vi "Convert From JSON Comp Format.vi"(8 "error in (no error)":errorcluster, 11 "input settings JSON":T1={"number of channels"=51200, "data justification"="", "endianness"="", "channel length"=5, "bit depth"=0, "frame clock rate"=0.0, "bit clock edge sync"="", "master clock souce"="", "master clock rate"=0.0, "logic level"="", "frame sync edge for channel 0"="", "Channel 0 Offset"=0}) -> (0 "error out":errorcluster, 3 "input settings":T2={"number of channels"=51200, "data justification"=enum."Right Justified", "endianness"=enum."MSB First", "channel length"=0, "bit depth"=0, "frame clock rate"=0.0, "bit clock edge sync"=enum."Falling", "master clock source"=enum."Internal", "master clock rate"=0.0, "Logic Level"=enum."1.2 V", "frame sync edge for channel 0"=enum."Rising", "Channel 0 Offset"=0})   [LabVIEW 2022 SP3, in "Digital Serial Input Settings.lvlib"]
uses:
  Digital Serial Input Settings.lvlib
  controls/digital serial input settings.ctl
  <vilib>/PDM Acquisition Toolkit/shared/controls/PCM Data Justification.ctl
  <vilib>/PDM Acquisition Toolkit/shared/controls/PCM Bit Endianness.ctl
  <vilib>/PDM Acquisition Toolkit/shared/controls/Digital Edge.ctl
  controls/digital audio protocol/master clock source.ctl
  <vilib>/PDM Acquisition Toolkit/host/Classes/Session/Controls/Logic Levels.ctl
  digital serial input settings_json.ctl
  <vilib>/PDM Acquisition Toolkit/shared/PDM Shared.lvlib
  <vilib>/PDM Acquisition Toolkit/host/Classes/Session/DecoderSession.lvclass
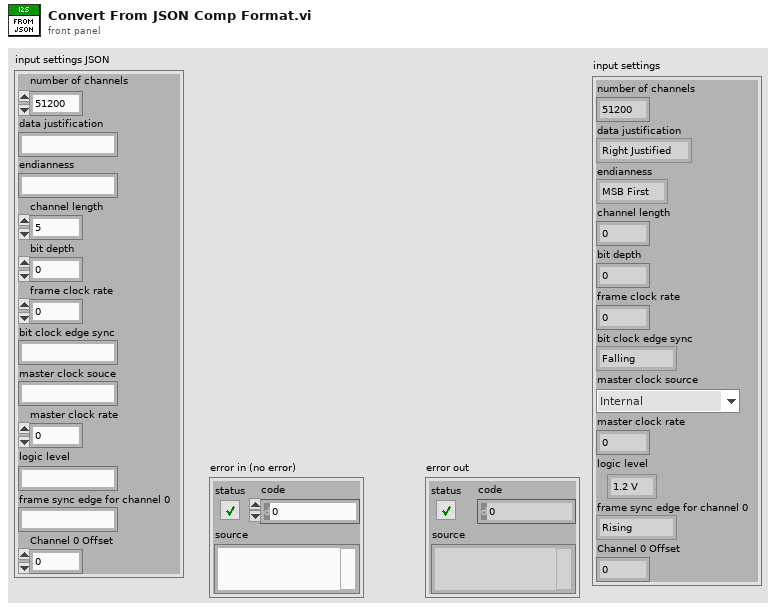
[diagram p1: front panel]
types:
  T1 = typedef "Digital Serial Input Settings.lvlib/digital serial input settings_json.ctl" = cluster{"number of channels":u32, "data justification":string, "endianness":string, "channel length":u32, "bit depth":u32, "frame clock rate":dbl, "bit clock edge sync":string, "master clock souce":string, "master clock rate":dbl, "logic level":string, "frame sync edge for channel 0":string, "Channel 0 Offset":u32}
  T2 = typedef "digital serial input settings.ctl" = cluster{"number of channels":u32, "data justification":T3, "endianness":T4, "channel length":u32, "bit depth":u32, "frame clock rate":dbl, "bit clock edge sync":T5, "master clock source":T6, "master clock rate":dbl, "Logic Level":T7, "frame sync edge for channel 0":T5, "Channel 0 Offset":u32}
  T3 = typedef "PDM Shared.lvlib/PCM Data Justification.ctl" = enum16{"Left Justified", "Right Justified"}
  T4 = typedef "PDM Shared.lvlib/PCM Bit Endianness.ctl" = enum16{"MSB First", "LSB First"}
  T5 = typedef "PDM Shared.lvlib/Digital Edge.ctl" = enum8{"Rising", "Falling"}
  T6 = typedef "master clock source.ctl" = enum32{"Internal", "External"}
  T7 = typedef "PDM Acquisition Class Library.lvlib/DecoderSession.lvclass/Logic Levels.ctl" = enum16{"3.3 V", "1.8 V", "1.2 V"}
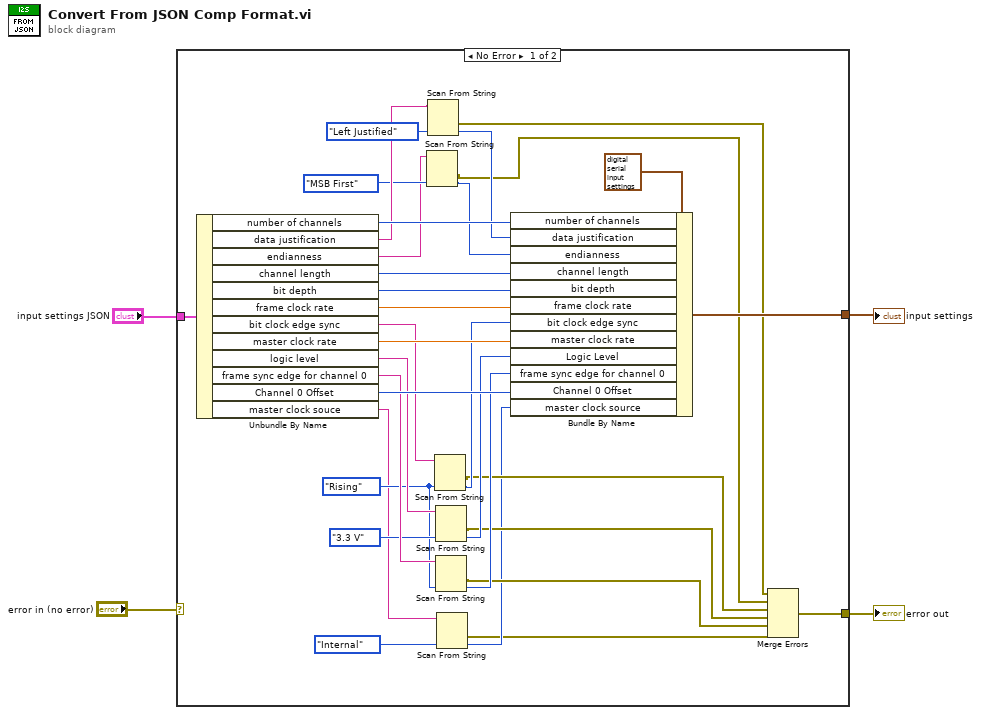
[diagram p0: block diagram]
diagram:
  n1 = case shown="No Error" "error in (no error)" {
    selector: "error in (no error)" -> [_ w38]
    tunnel: "input settings JSON" -> [w30 _]
    tunnel: [w29 _] -> w2
    tunnel: [w9 w38] -> w1
    frame No Error {
      w18 = Digital_Edge."Rising" ("bit clock edge sync")
      n2 = Unbundle By Name(w30) -> ("number of channels"=w37:u32, "data justification"=w28:string, "endianness"=w24:string, "channel length"=w36:u32, "bit depth"=w35:u32, "frame clock rate"=w34:dbl, "bit clock edge sync"=w22:string, "master clock rate"=w33:dbl, "logic level"=w21:string, "frame sync edge for channel 0"=w20:string, "Channel 0 Offset"=w32:u32, "master clock souce"=w8:string)
      n3 = Scan From String(input string=w24, default 1=PCM_Bit_Endianness."MSB First" ("endianness")) -> (error out=w13:errorcluster, output 1=w23:T4)  [unwired: 3 in, 2 out]
      n4 = Scan From String(input string=w28, default 1=PCM_Data_Justification."Left Justified" ("data justification")) -> (error out=w14:errorcluster, output 1=w26:T3)  [unwired: 3 in, 2 out]
      n5 = Scan From String(input string=w22, default 1=w18) -> (error out=w12:errorcluster, output 1=w17:T5)  [unwired: 3 in, 2 out]
      n6 = Scan From String(input string=w21, default 1=Logic_Levels."3.3 V" ("Logic Level")) -> (error out=w11:errorcluster, output 1=w16:T7)  [unwired: 3 in, 2 out]
      n7 = Scan From String(input string=w20, default 1=w18) -> (error out=w10:errorcluster, output 1=w15:T5)  [unwired: 3 in, 2 out]
      n8 = Scan From String(input string=w8, default 1=master_clock_source."Internal" ("master clock source")) -> (error out=w5:errorcluster, output 1=w6:T6)  [unwired: 3 in, 2 out]
      n9 = Bundle By Name(cluster=T2 {"number of channels"=0, "data justification"=enum."Left Justified", "endianness"=enum."LSB First", "channel length"=0, "bit depth"=0, "frame clock rate"=0.0, "bit clock edge sync"=enum."Falling", "master clock source"=enum."Internal", "master clock rate"=0.0, "Logic Level"=enum."1.2 V", "frame sync edge for channel 0"=enum."Rising", "Channel 0 Offset"=0} ("digital serial input settings"), "number of channels"=w37, "data justification"=w26, "endianness"=w23, "channel length"=w36, "bit depth"=w35, "frame clock rate"=w34, "bit clock edge sync"=w17, "master clock rate"=w33, "Logic Level"=w16, "frame sync edge for channel 0"=w15, "Channel 0 Offset"=w32, "master clock source"=w6) -> (w29:T2)
      n10 = Merge Errors(w14, w13, w12, w11, w10, w5) -> (w9:errorcluster)
    }
    frame Error {
    }
  }
  "input settings" <- w2
  "error out" <- w1
